vi "Washing.vi"(8 "Error In":errorcluster, 11 "time target (s)":dbl) -> (0 "Error Out":errorcluster)   [LabVIEW 2017]
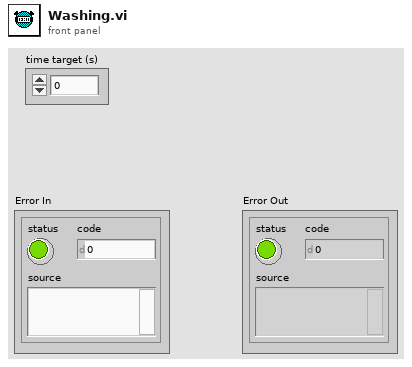
[diagram p1: front panel]
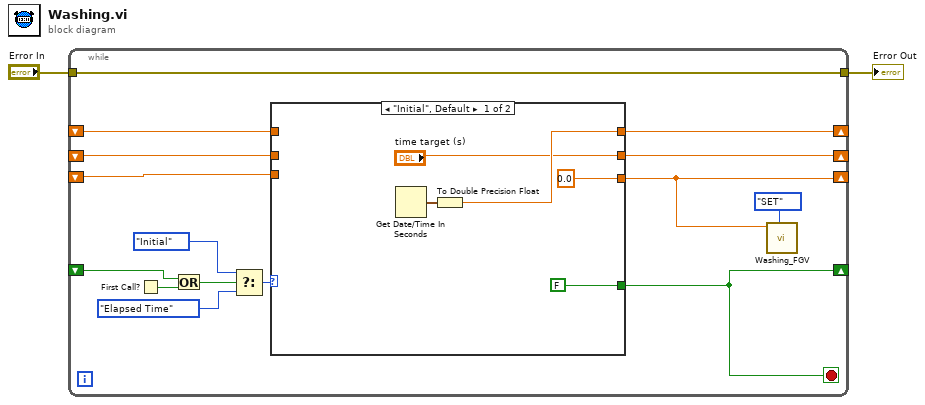
[diagram p0: block diagram]
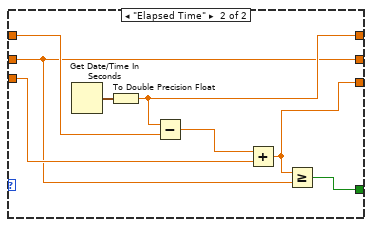
[diagram p2: hidden frame]
diagram:
  n1 = while {
    tunnel: [w17] -> w2
    tunnel: "Error In" -> [w17]
    shift-right: [w8] -> _
    shift-left: _ -> [w11]
    shift-right: [w7] -> _
    shift-left: _ -> [w10]
    shift-right: [w3] -> _
    shift-left: _ -> [w9]
    shift-right: [w5] -> _
    shift-left: _ -> [w6]
    stop <- w5 stop-if-true
    n2 = First Call?() -> (First Call?: T/F=w13:bool)
    n3 = Or(x=w6, y=w13) -> (x .or. y?=w14:bool)
    n4 = Select(t=enum16{"Initial", "Elapsed Time"}."Initial", s=w14, f=enum16{"Initial", "Elapsed Time"}."Elapsed Time") -> (s? t:f=w15:enum16{"Initial", "Elapsed Time"})
    n5 = case shown="\"Initial\", Default" w15 {
      tunnel: ["time target (s)" w25] -> w7
      tunnel: w10 -> [_ w25]
      tunnel: [w20 w28] -> w8
      tunnel: w11 -> [_ w29]
      tunnel: [0.0 w24] -> w3
      tunnel: w9 -> [_ w27]
      tunnel: [FALSE w26] -> w5
      frame "Initial", Default {
        n6 = Get Date/Time In Seconds() -> (seconds since 1Jan1904=w21:timestamp)
        n7 = To Double Precision Float(number=w21) -> (double precision float=w20:dbl)
      }
      frame "Elapsed Time" {
        n8 = Get Date/Time In Seconds() -> (seconds since 1Jan1904=w30:timestamp)
        n9 = To Double Precision Float(number=w30) -> (double precision float=w28:dbl)
        n10 = Subtract(x=w28, y=w29) -> (x-y=w23:dbl)
        n11 = Add(x=w23, y=w27) -> (x+y=w24:dbl)
        n12 = Greater Or Equal?(x=w24, y=w25) -> (x >= y?=w26:bool)
      }
    }
    n13 = call "Washing_FGV.vi"("Command"=enum16{"SET", "GET"}."SET", "Elased_Time(s)"=w3) -> ()  [unwired: 8 in, 2 out]
  }
  "Error Out" <- w2
